vi "Apply New Library Tools-Options Settings.vi"(8 "error in (no error)":errorcluster, 11 "Library Refnum":refnum<vi>) -> (0 "error out":errorcluster, 3 "dup Library Refnum":refnum<vi>)   [LabVIEW 2020]
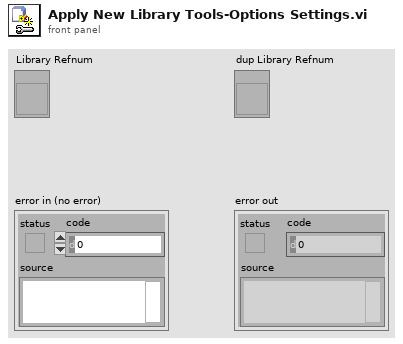
[diagram p1: front panel]
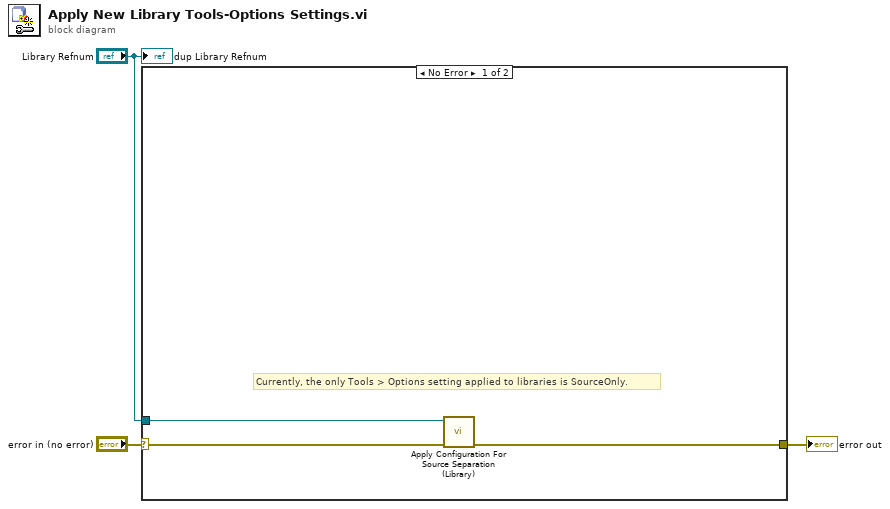
[diagram p0: block diagram]
diagram:
  n1 = case shown="No Error" "error in (no error)" {
    selector: "error in (no error)" -> [w6 w7]
    tunnel: [w5 w7] -> w2
    tunnel: "Library Refnum" -> [w4 _]
    frame No Error {
      # "Currently, the only Tools > Options setting applied to libraries is SourceOnly."
      n2 = call <vilib>:"Apply Configuration For Source Separation (Library).vi"("error in (no error)"=w6, "Library in"=w4) -> ("error out"=w5:errorcluster)  [unwired: 8 in, 1 out]
    }
    frame Error {
    }
  }
  "error out" <- w2
  "dup Library Refnum" <- "Library Refnum"
